vi "WhileLoopExample.vi"() -> ()   [LabVIEW 2020]
panel:
  out "Liczba obrotów pętli -1":i32
  out "Wszystkie liczby losowe \n>1,5":dbl[](array[numeric])
  in  "Error In":errorcluster
  out "Wszystkie liczby losowe":dbl[](array[numeric])
  in  "Stop":bool
  out "Wykres liczb losowych":dbl(graph)
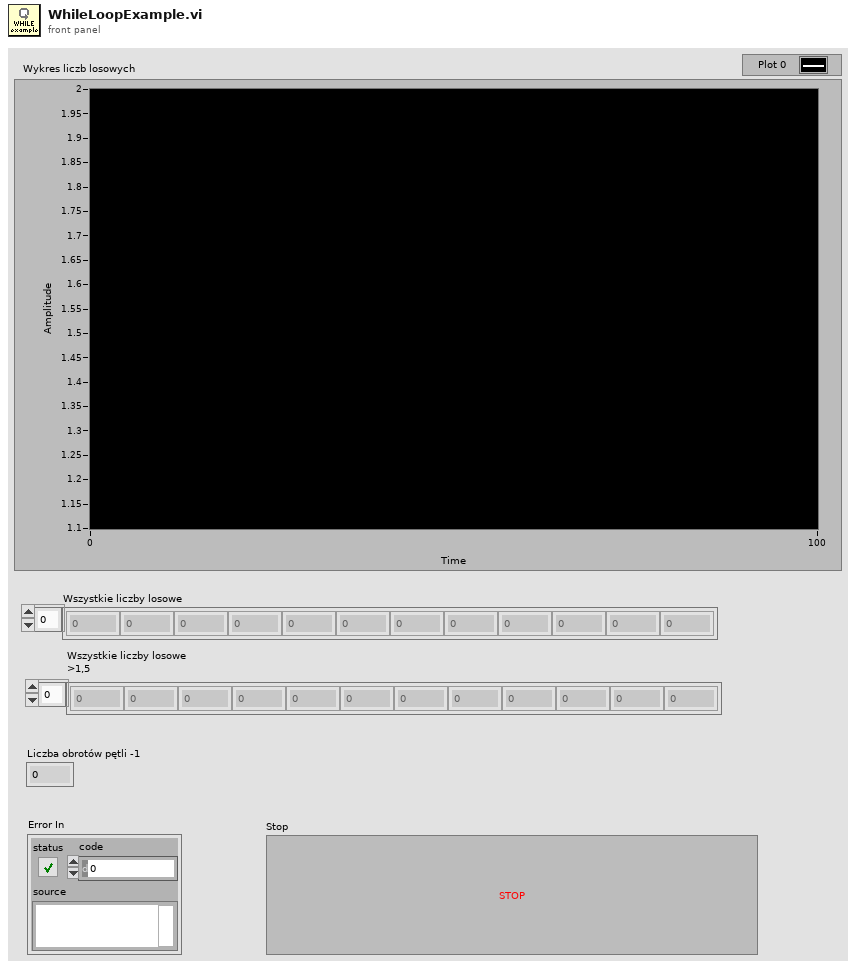
[diagram p1: front panel]
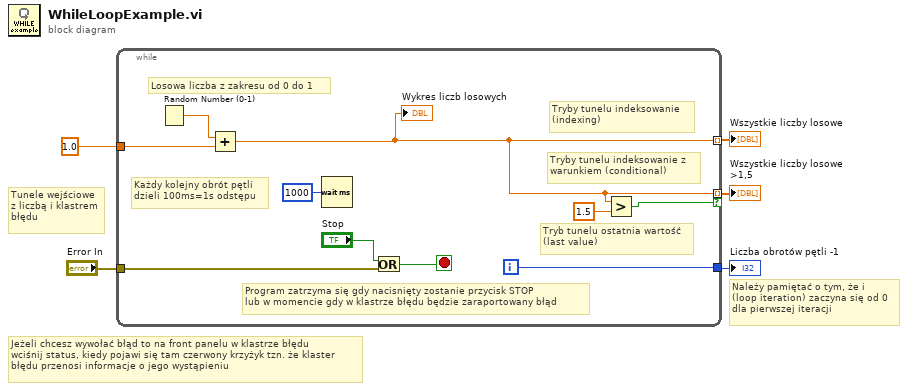
[diagram p0: block diagram]
diagram:
  # "Jeżeli chcesz wywołać błąd to na front panelu w klastrze błędu\nwciśnij status, kiedy pojawi się tam czerwony krzyżyk tzn. że klaster\nbłędu przenosi informacje o jego wystąpieniu"
  # "Tunele wejściowe\nz liczbą i klastrem\nbłędu"
  # "Należy pamiętać o tym, że i \n(loop iteration) zaczyna się od 0\ndla pierwszej iteracji"
  n1 = while {
    tunnel: 1.0 -> [w13]
    tunnel: [w9] -> w4 mode=indexing
    tunnel: "Error In" -> [w10]
    tunnel: [w9] -> w2 mode=indexing if=w7
    tunnel: [w6] -> w1
    i -> [w6]
    stop <- w11 stop-if-true
    # "Losowa liczba z zakresu od 0 do 1"
    # "Tryb tunelu ostatnia wartość\n(last value)"
    # "Tryby tunelu indeksowanie z\nwarunkiem (conditional)"
    # "Tryby tunelu indeksowanie\n(indexing)"
    # "Każdy kolejny obrót pętli \ndzieli 100ms=1s odstępu"
    # "Program zatrzyma się gdy nacisnięty zostanie przycisk STOP\nlub w momencie gdy w klastrze błędu będzie zaraportowany błąd"
    n2 = Random Number (0-1)() -> (number: 0 to 1=w14:dbl)
    n3 = Add(x=w14, y=w13) -> (x+y=w9:dbl)
    "Wykres liczb losowych" <- w9
    n4 = Wait (ms)(milliseconds to wait=u32 1000) -> ()  [unwired: 1 out]
    n5 = Or(x="Stop", y=w10) -> (x .or. y?=w11:bool)
    n6 = Greater?(x=w9, y=1.5) -> (0:w7:bool)
  }
  "Wszystkie liczby losowe" <- w4
  "Wszystkie liczby losowe \n>1,5" <- w2
  "Liczba obrotów pętli -1" <- w1
